vi "Defragment Tdms File.vi"() -> ()   [LabVIEW 2020]
panel:
  in  "file path":path
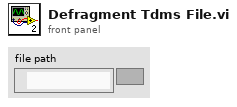
[diagram p1: front panel]
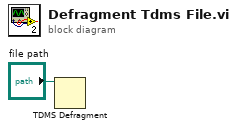
[diagram p0: block diagram]
diagram:
  n1 = TDMS Defragment(7:"file path") -> ()  [unwired: 1 in, 1 out]
